vi "inficon_slow.vi"(3 "error out":errorcluster, 4 "string to write":string="PR1", 5 "VISA resource name":refnum<visa-resource-name>="COM1") -> (0 "error out 2":errorcluster, 1 "read buffer 2":string, 2 "VISA resource name 2":refnum<visa-resource-name>)   [LabVIEW 2015]
panel:
  out "Serial Settings:Number of Bytes at Serial Port 2":u32
  out "Serial Settings:Number of Bytes at Serial Port":u32
  out "buffer lu":string
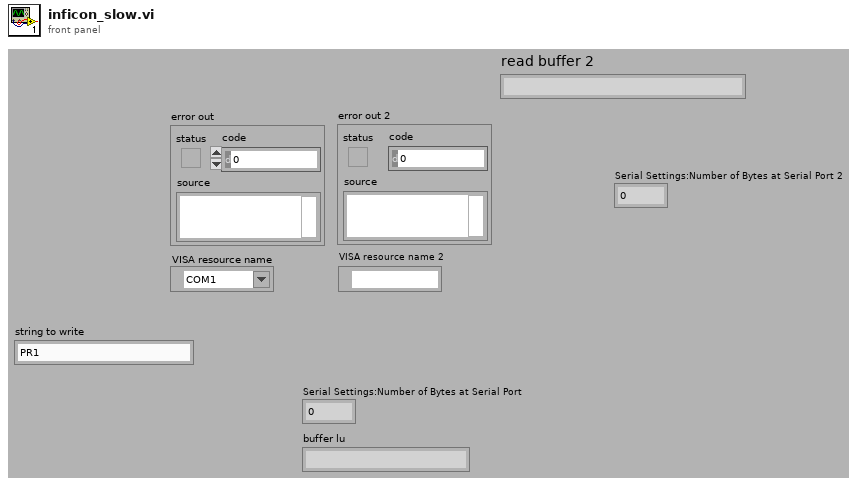
[diagram p1: front panel]
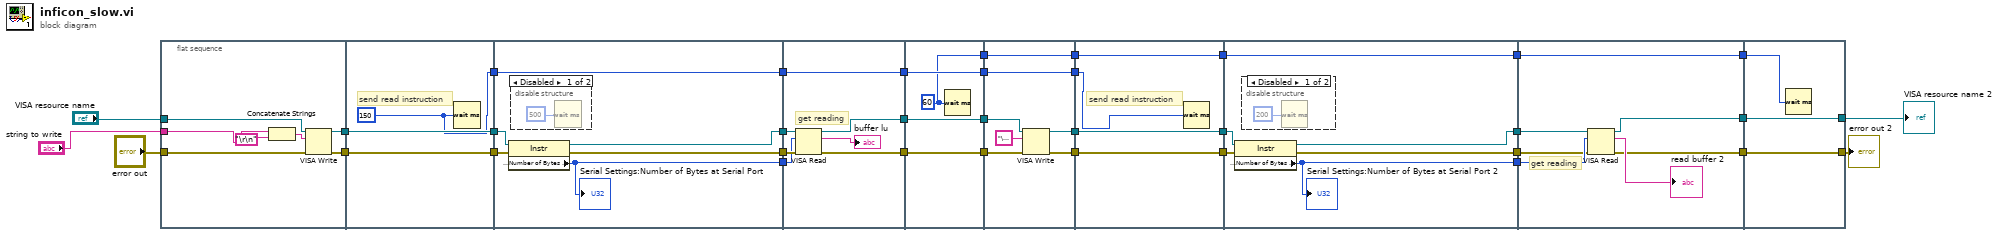
[diagram p0: block diagram]
diagram:
  n1 = flat-sequence {
    tunnel: [w41] -> w31
    tunnel: [w40] -> w29
    tunnel: "VISA resource name" -> [w42]
    tunnel: "error out" -> [w37]
    tunnel: "string to write" -> [w36]
    tunnel: w31 -> [w45]
    tunnel: [w45] -> w30
    tunnel: w29 -> [w44]
    tunnel: [w44] -> w28
    tunnel: [w43] -> w6
    tunnel: w30 -> [w51]
    tunnel: w28 -> [w50]
    tunnel: [w49] -> w34
    tunnel: [w48] -> w33
    tunnel: [w47] -> w32
    tunnel: [w46] -> w7
    tunnel: w6 -> [w46]
    tunnel: w34 -> [w59]
    tunnel: w33 -> [w58]
    tunnel: w32 -> [w55]
    tunnel: [w57] -> w19
    tunnel: [w56] -> w17
    tunnel: [w53] -> w8
    tunnel: w7 -> [w53]
    tunnel: w19 -> [w63]
    tunnel: [w63] -> w18
    tunnel: w17 -> [w62]
    tunnel: [w62] -> w16
    tunnel: [w61] -> w9
    tunnel: w8 -> [w61]
    tunnel: [w60] -> w1
    tunnel: w18 -> [w70]
    tunnel: w16 -> [w69]
    tunnel: [w68] -> w27
    tunnel: [w67] -> w25
    tunnel: [w65] -> w10
    tunnel: w9 -> [w65]
    tunnel: [w64] -> w2
    tunnel: w1 -> [w64]
    tunnel: w27 -> [w73]
    tunnel: [w74] -> w26
    tunnel: w25 -> [w74]
    tunnel: [w73] -> w24
    tunnel: w10 -> [w72]
    tunnel: [w71] -> w3
    tunnel: w2 -> [w71]
    tunnel: w26 -> [w80]
    tunnel: w24 -> [w79]
    tunnel: [w78] -> w23
    tunnel: [w77] -> w22
    tunnel: [w76] -> w21
    tunnel: [w75] -> w4
    tunnel: w3 -> [w75]
    tunnel: w23 -> [w88]
    tunnel: w22 -> [w87]
    tunnel: w21 -> [w86]
    tunnel: [w85] -> w15
    tunnel: [w83] -> w13
    tunnel: [w82] -> w5
    tunnel: w4 -> [w82]
    tunnel: [w91] -> w20
    tunnel: w15 -> [w91]
    tunnel: w13 -> [w90]
    tunnel: [w90] -> w12
    tunnel: w5 -> [w89]
    frame #0 {
      n2 = Concatenate Strings(w36, "\r\n") -> (w38:string)
      n3 = VISA Write(VISA resource name=w42, write buffer=w38, error in (no error)=w37) -> (VISA resource name out=w41:refnum<visa-resource-name>, error out=w40:errorcluster)  [unwired: 1 out]
    }
    frame #1 {
      w43 = u32 150 ("milliseconds to wait")
      # "send read instruction"
      n4 = Wait (ms)(milliseconds to wait=w43) -> ()  [unwired: 1 out]
    }
    frame #2 {
      n5 = property class="Instr"(reference=w51, error in=w50) -> (reference out=w49:refnum<visa-resource-name>, error out=w48:errorcluster, "Serial Settings:Number of Bytes at Serial Port"=w47:u32)
      "Serial Settings:Number of Bytes at Serial Port" <- w47
      n6 = disable-structure shown="Disabled" {
        frame Disabled {
          n7 = Wait (ms)(milliseconds to wait=u32 500) -> ()  [unwired: 1 out]
        }
        frame Enabled {
        }
      }
    }
    frame #3 {
      # "get reading"
      n8 = VISA Read(VISA resource name=w59, byte count=w55, error in (no error)=w58) -> (VISA resource name out=w57:refnum<visa-resource-name>, read buffer=→"buffer lu":string, error out=w56:errorcluster)  [unwired: 1 out]
    }
    frame #4 {
      w60 = u32 60 ("milliseconds to wait")
      n9 = Wait (ms)(milliseconds to wait=w60) -> ()  [unwired: 1 out]
    }
    frame #5 {
      n10 = VISA Write(VISA resource name=w70, write buffer="\u0005" ("string"), error in (no error)=w69) -> (VISA resource name out=w68:refnum<visa-resource-name>, error out=w67:errorcluster)  [unwired: 1 out]
    }
    frame #6 {
      # "send read instruction"
      n11 = Wait (ms)(milliseconds to wait=w72) -> ()  [unwired: 1 out]
    }
    frame #7 {
      n12 = property class="Instr"(reference=w79, error in=w80) -> (reference out=w77:refnum<visa-resource-name>, error out=w76:errorcluster, "Serial Settings:Number of Bytes at Serial Port"=w78:u32)
      "Serial Settings:Number of Bytes at Serial Port 2" <- w78
      n13 = disable-structure shown="Disabled" {
        frame Disabled {
          n14 = Wait (ms)(milliseconds to wait=u32 200) -> ()  [unwired: 1 out]
        }
        frame Enabled {
        }
      }
    }
    frame #8 {
      # "get reading"
      n15 = VISA Read(VISA resource name=w87, byte count=w88, error in (no error)=w86) -> (VISA resource name out=w85:refnum<visa-resource-name>, read buffer=→"read buffer 2":string, error out=w83:errorcluster)  [unwired: 1 out]
    }
    frame #9 {
      n16 = Wait (ms)(milliseconds to wait=w89) -> ()  [unwired: 1 out]
    }
  }
  "VISA resource name 2" <- w20
  "error out 2" <- w12
